vi "headingOnWP.vi"(9 "psi":dbl, 10 "p_d":dbl[](array[numeric]), 11 "pt":dbl[](array[numeric])) -> (2 "e_psi":dbl, 4 "psi_d":dbl)   [LabVIEW 2014]
uses:
  <vilib>/imath/engines/lvmath2/RunTimeEngine/BuiltInFunctions/atan2/NIMS_atan2.vi
  <instcachedir>/0/NIMS_atan2_A91AA4A7D42247EDBE8F76DB99AF04A4.lvgen/NIMS_atan2_A91AA4A7D42247EDBE8F76DB99AF04A4_000.vi
  <vilib>/imath/engines/lvmath2/RunTimeEngine/BuiltInFunctions/abs/NIMS_abs(signed).vi
  <instcachedir>/0/NIMS_abs(signed)_C4FCB8E6058B49B797C7C8D53CA5F6EC.lvgen/NIMS_abs(signed)_C4FCB8E6058B49B797C7C8D53CA5F6EC_000.vi
  <vilib>/imath/engines/lvmath2/RunTimeEngine/NodeEndStatement/NIMS_NodeEndStatement_Output.vi
  <instcachedir>/0/NIMS_NodeEndStatement_Output_53EC0D466D134D7ABD903AC30B43404B.lvgen/NIMS_NodeEndStatement_Output_53EC0D466D134D7ABD903AC30B43404B_001.vi
  <vilib>/imath/engines/lvmath2/RunTimeEngine/ErrorHandling/NIMS_Finalize Error.vi
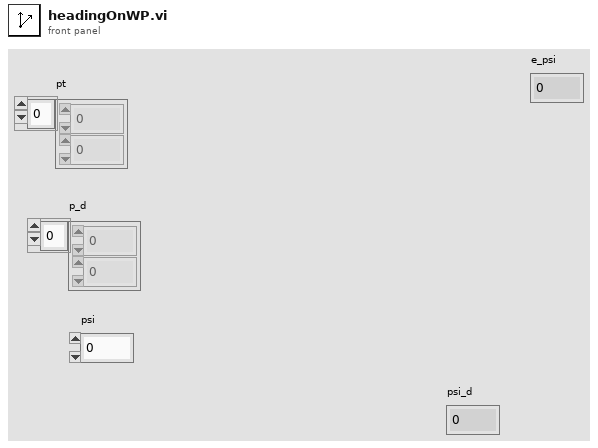
[diagram p1: front panel]
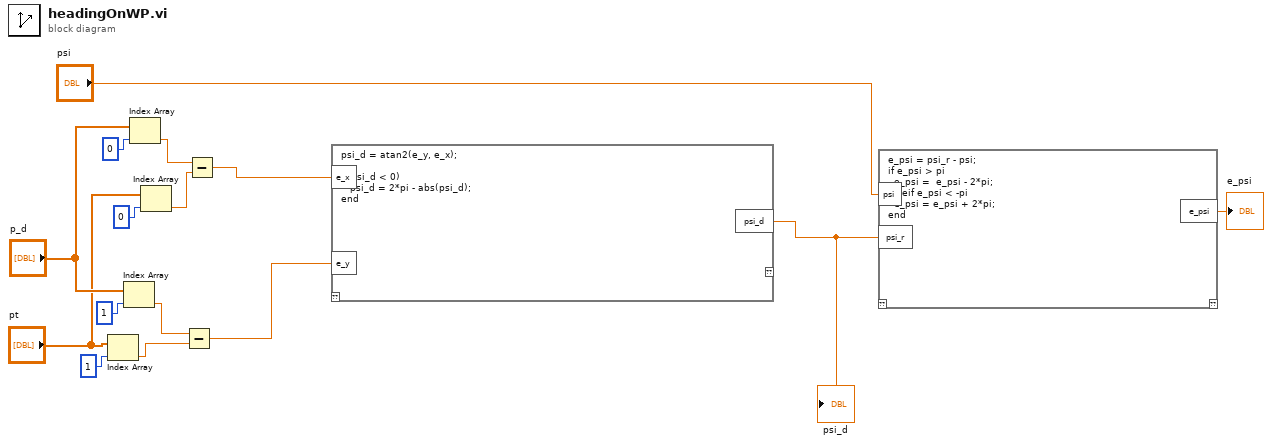
[diagram p0: block diagram]
diagram:
  n1 = Index Array(array="pt", index=1) -> (element=w7:dbl)
  n2 = Index Array(array="p_d", index=1) -> (element=w11:dbl)
  n3 = Index Array(array="p_d", index=0) -> (element=w12:dbl)
  n4 = Index Array(array="pt", index=0) -> (element=w6:dbl)
  n5 = Subtract(x=w11, y=w7) -> (x-y=w4:dbl)
  n6 = Subtract(x=w12, y=w6) -> (x-y=w5:dbl)
  n7 = mathscript code="psi_d = atan2(e_y, e_x);\n\nif(psi_d < 0)\n   psi_d = 2*pi - abs(psi_d);\nend"("e_x"=w5, "e_y"=w4) -> ("psi_d"=w2:dbl)  [unwired: 1 in, 1 out]
  "psi_d" <- w2
  n8 = mathscript code="e_psi = psi_r - psi;\nif e_psi > pi\n  e_psi =  e_psi - 2*pi;\nelseif e_psi < -pi\n  e_psi = e_psi + 2*pi;\nend"("psi"="psi", "psi_r"=w2) -> ("e_psi"=→"e_psi":dbl)  [unwired: 1 in, 1 out]
